vi "EngineeringTool.vi"() -> ()   [LabVIEW 2014]
uses:
  EngineeringGlobals.vi
panel:
  out "Connected":bool
  in  "Close":bool
  in  "Tab Control":enum32{"General", "ARC", "Headers", "Misc"}(tab)
  in  "DSP Code":bool
  in  "Detector":bool
  in  "Temperatures":bool
  in  "Test Shutter":bool
  in  "Manual Commands":bool
  in  "Clear Detector":bool
  in  "Reset Command":bool
  in  "Test Fibers":bool
  in  "Read/Write DSP Memory":bool
  in  "Start Idle Clocks":bool
  in  "Stop Idle Clocks":bool
  in  "Digital I/O":bool
  in  "GetControllerHeader":bool
  in  "GetInstrumentHeader":bool
  in  "GetTelescopeHeader":bool
  out "Server":string
  out "Port":i32
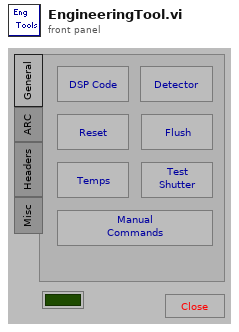
[diagram p1: front panel]
types:
  T1 = typedef "LVRectTypeDef.ctl" = cluster{"Left":i16, "Top":i16, "Right":i16, "Bottom":i16}
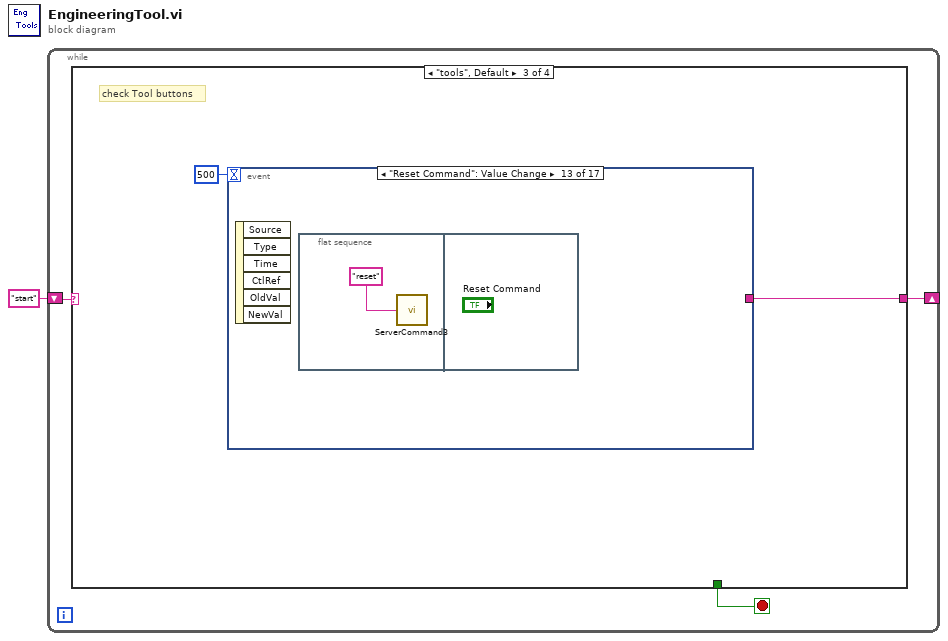
[diagram p0: block diagram]
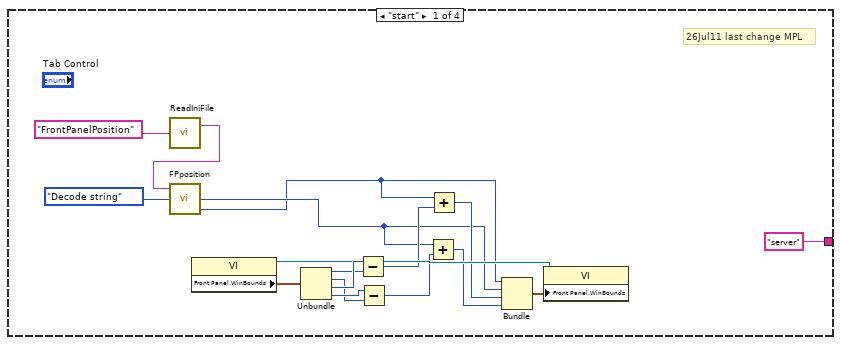
[diagram p2: hidden frame]
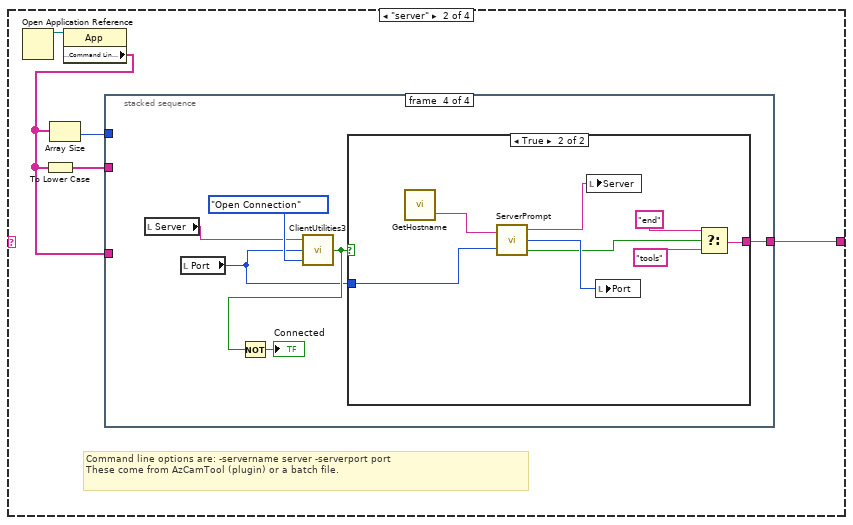
[diagram p3: hidden frame]
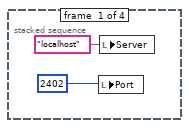
[diagram p4: hidden frame]
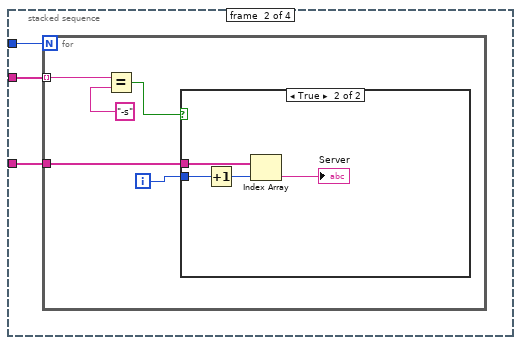
[diagram p5: hidden frame]
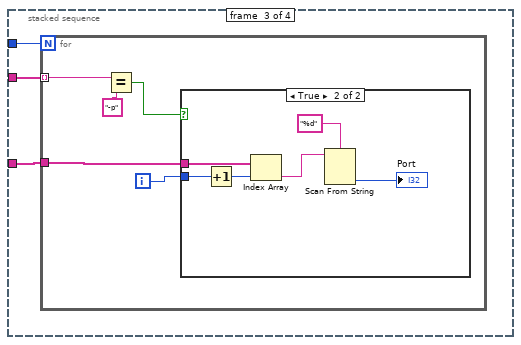
[diagram p7: hidden frame]
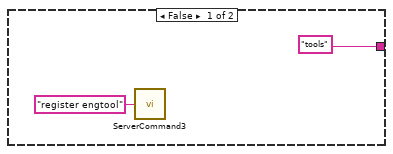
[diagram p9: hidden frame]
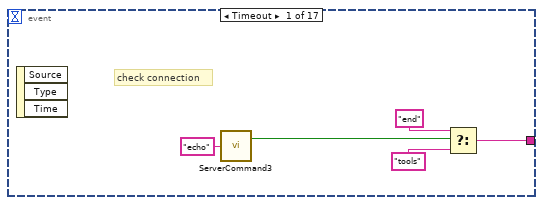
[diagram p10: hidden frame]
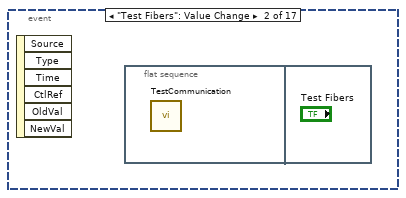
[diagram p11: hidden frame]
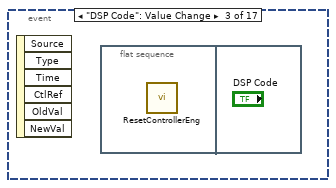
[diagram p12: hidden frame]
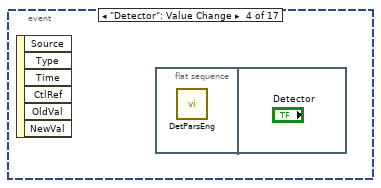
[diagram p13: hidden frame]
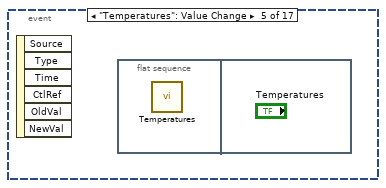
[diagram p14: hidden frame]
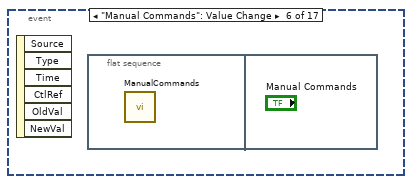
[diagram p15: hidden frame]
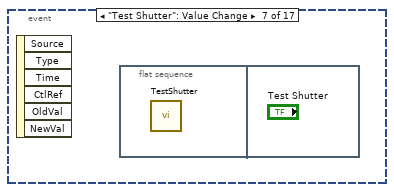
[diagram p16: hidden frame]
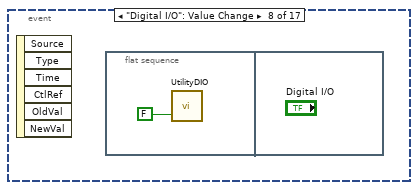
[diagram p17: hidden frame]
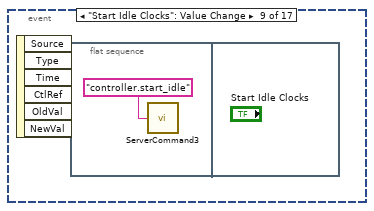
[diagram p18: hidden frame]
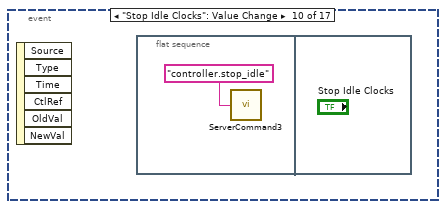
[diagram p19: hidden frame]
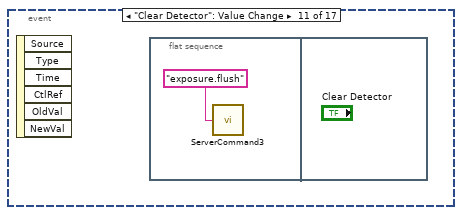
[diagram p20: hidden frame]
diagram:
  n1 = while {
    shift-right: [w3] -> _
    shift-left: "start" -> [w4]
    stop <- w2 stop-if-true
    n2 = case shown="\"tools\", Default" w4 {
      tunnel: ["server" w22 w72 _] -> w3
      tunnel: [_ _ _ TRUE] -> w2
      frame "start" {
        # "26Jul11 last change MPL"
        n3 = call "ReadIniFile.vi"("key"="FrontPanelPosition") -> ("value"=w5:string)  [unwired: 1 out]
        n4 = call "FPposition.vi"("Action"=enum16{"Make string", "Decode string"}."Decode string", "String In"=w5) -> ("left"=w7:i32, "top"=w8:i32)  [unwired: 1 in, 1 out]
        n5 = property class="VI"() -> (reference out=w15:refnum<vi>, "Front Panel.WinBounds"=w20:T1)  [unwired: 2 in, 1 out]
        n6 = Unbundle(w20) -> ("Left"=w18:i16, "Top"=w16:i16, "Right"=w19:i16, "Bottom"=w17:i16)
        n7 = Subtract(x=w19, y=w18) -> (x-y=w11:i16)
        n8 = Subtract(x=w17, y=w16) -> (x-y=w10:i16)
        n9 = Add(x=w8, y=w10) -> (x+y=w12:i32)
        n10 = Add(x=w7, y=w11) -> (x+y=w13:i32)
        n11 = Bundle("left"=w7, "top"=w8, w13, w12) -> (w14:cluster{"left":i32, "top":i32, i32, i32})  [unwired: 1 in]
        n12 = property class="VI"(reference=w15, "Front Panel.WinBounds"=w14) -> ()  [unwired: 1 in, 2 out]
      }
      frame "server" {
        # "Command line options are: -servername server -serverport port\nThese come from AzCamTool (plugin) or a batch file."
        n13 = Open Application Reference() -> (3:w26:refnum<vi>)  [unwired: 4 in, 1 out]
        n14 = property class="App"(reference=w26) -> ("Application:Command Line Arguments"=w24:string[])  [unwired: 1 in, 2 out]
        n15 = To Lower Case(string=w24) -> (all lower case string=w25:string[])
        n16 = Array Size(array=w24) -> (size(s)=w23:i32)
        n17 = stacked-sequence {
          tunnel: w24 -> [_ w30 w42 _]
          tunnel: w25 -> [_ w31 w43 _]
          tunnel: w23 -> [_ w29 w41 _]
          tunnel: [_ _ _ w58] -> w22
          frame #0 {
            n18 = local write "Port"(u16 2402 ("AzCamServer Port")) -> ()
            n19 = local write "Server"("localhost" ("Server")) -> ()
          }
          frame #1 {
            n20 = for {
              N: w29 -> [_]
              tunnel: w31 -> [w34] mode=indexing
              tunnel: w30 -> [w33]
              i -> [w32]
              n21 = Equal?(x=w34, y="-s" ("x")) -> (x = y?=w35:bool)
              n22 = case shown="True" w35 {
                tunnel: w33 -> [_ w39]
                tunnel: w32 -> [_ w38]
                frame False {
                }
                frame True {
                  n23 = Increment(x=w38) -> (x+1=w40:i32)
                  n24 = Index Array(array=w39, index=w40) -> (element=→"Server":string)
                }
              }
            }
          }
          frame #2 {
            n25 = for {
              N: w41 -> [_]
              tunnel: w43 -> [w46] mode=indexing
              tunnel: w42 -> [w45]
              i -> [w44]
              n26 = Equal?(x=w46, y="-p" ("x")) -> (x = y?=w47:bool)
              n27 = case shown="True" w47 {
                tunnel: w45 -> [_ w53]
                tunnel: w44 -> [_ w52]
                frame False {
                }
                frame True {
                  n28 = Increment(x=w52) -> (x+1=w54:i32)
                  n29 = Index Array(array=w53, index=w54) -> (element=w51:string)
                  n30 = Scan From String(format string="%d", input string=w51) -> (output 1=→"Port":i32)  [unwired: 3 in, 3 out]
                }
              }
            }
          }
          frame #3 {
            n31 = local read "Server"() -> (w59:string)
            n32 = local read "Port"() -> (w55:i32)
            n33 = call "ClientUtilities3.vi"("Action"=enum16{"Open Connection"}."Open Connection", "ServerPort"=w55, "ServerName"=w59) -> ("Error"=w57:bool)
            n34 = Not(x=w57) -> (.not. x?=→"Connected":bool)
            n35 = case shown="True" w57 {
              tunnel: ["tools" w65] -> w58
              tunnel: w55 -> [_ w63]
              frame False {
                n36 = call "ServerCommand3.vi"("Command"="register engtool") -> ()  [unwired: 2 out]
              }
              frame True {
                n37 = call "GetHostname.vi"() -> ("Name"=w68:string)  [unwired: 1 in, 1 out]
                n38 = call "ServerPrompt.vi"("AzCam Hostname"=w68, "Port"=w63) -> ("ServerOut"=w70:string, "Port Out"=w69:u16, "Error"=w64:bool)
                n39 = local write "Server"(w70) -> ()
                n40 = local write "Port"(w69) -> ()
                n41 = Select(t="end", s=w64, f="tools") -> (s? t:f=w65:string)
              }
            }
          }
        }
      }
      frame "tools", Default {
        # "check Tool buttons"
        n42 = event shown="[12] \"Reset Command\": Value Change" {
          selector: _ -> [_ _ _ _ _ _ _ _ _ _ _ _ _ _ _ _ _]
          dyn-events: _ -> [_ _ _ _ _ _ _ _ _ _ _ _ _ _ _ _ _]
          timeout: 500 -> [_ _ _ _ _ _ _ _ _ _ _ _ _ _ _ _ _]
          tunnel: [w77 _ _ _ _ _ _ _ _ _ _ _ _ _ _ _ "end"] -> w72
          event Timeout {
            # "check connection"
            n43 = event-data() -> ()  [unwired: 1 in, 3 out]
            n44 = call "ServerCommand3.vi"("Command"="echo") -> ("Error"=w73:bool)  [unwired: 1 out]
            n45 = Select(t="end", s=w73, f="tools") -> (s? t:f=w77:string)
          }
          event "Test Fibers": Value Change {
            n46 = event-data() -> ()  [unwired: 1 in, 6 out]
            n47 = flat-sequence {
              frame #0 {
                n48 = call "TestCommunication.vi"() -> ()  [unwired: 1 in]
              }
              frame #1 {
              }
            }
          }
          event "DSP Code": Value Change {
            n49 = event-data() -> ()  [unwired: 1 in, 6 out]
            n50 = flat-sequence {
              frame #0 {
                n51 = call "ResetControllerEng.vi"() -> ()  [unwired: 1 in, 1 out]
              }
              frame #1 {
              }
            }
          }
          event "Detector": Value Change {
            n52 = event-data() -> ()  [unwired: 1 in, 6 out]
            n53 = flat-sequence {
              frame #0 {
                n54 = call "DetParsEng.vi"() -> ()  [unwired: 2 in]
              }
              frame #1 {
              }
            }
          }
          event "Temperatures": Value Change {
            n55 = event-data() -> ()  [unwired: 1 in, 6 out]
            n56 = flat-sequence {
              frame #0 {
                n57 = call "Temperatures.vi"() -> ()  [unwired: 2 in, 1 out]
              }
              frame #1 {
              }
            }
          }
          event "Manual Commands": Value Change {
            n58 = event-data() -> ()  [unwired: 1 in, 6 out]
            n59 = flat-sequence {
              frame #0 {
                n60 = call "ManualCommands.vi"() -> ()  [unwired: 1 in, 1 out]
              }
              frame #1 {
              }
            }
          }
          event "Test Shutter": Value Change {
            n61 = event-data() -> ()  [unwired: 1 in, 6 out]
            n62 = flat-sequence {
              frame #0 {
                n63 = call "TestShutter.vi"() -> ()  [unwired: 1 in]
              }
              frame #1 {
              }
            }
          }
          event "Digital I/O": Value Change {
            n64 = event-data() -> ()  [unwired: 1 in, 6 out]
            n65 = flat-sequence {
              frame #0 {
                n66 = call "UtilityDIO.vi"("Immediate"=FALSE) -> ()  [unwired: 1 in, 1 out]
              }
              frame #1 {
              }
            }
          }
          event "Start Idle Clocks": Value Change {
            n67 = event-data() -> ()  [unwired: 1 in, 6 out]
            n68 = flat-sequence {
              frame #0 {
                n69 = call "ServerCommand3.vi"("Command"="controller.start_idle") -> ()  [unwired: 2 out]
              }
              frame #1 {
              }
            }
          }
          event "Stop Idle Clocks": Value Change {
            n70 = event-data() -> ()  [unwired: 1 in, 6 out]
            n71 = flat-sequence {
              frame #0 {
                n72 = call "ServerCommand3.vi"("Command"="controller.stop_idle") -> ()  [unwired: 2 out]
              }
              frame #1 {
              }
            }
          }
          event "Clear Detector": Value Change {
            n73 = event-data() -> ()  [unwired: 1 in, 6 out]
            n74 = flat-sequence {
              frame #0 {
                n75 = call "ServerCommand3.vi"("Command"="exposure.flush") -> ()  [unwired: 2 out]
              }
              frame #1 {
              }
            }
          }
          event "Read/Write DSP Memory": Value Change {
            n76 = event-data() -> ()  [unwired: 1 in, 6 out]
            n77 = flat-sequence {
              frame #0 {
                n78 = call "DSPMemory.vi"() -> ()  [unwired: 1 in]
              }
              frame #1 {
              }
            }
          }
          event "Reset Command": Value Change {
            n79 = event-data() -> ()  [unwired: 1 in, 6 out]
            n80 = flat-sequence {
              frame #0 {
                n81 = call "ServerCommand3.vi"("Command"="reset") -> ()  [unwired: 2 out]
              }
              frame #1 {
              }
            }
          }
          event "GetTelescopeHeader": Value Change {
            n82 = event-data() -> ()  [unwired: 1 in, 6 out]
            n83 = flat-sequence {
              frame #0 {
                n84 = call "TelescopeHeader.vi"() -> ()  [unwired: 1 in]
              }
              frame #1 {
              }
            }
          }
          event "GetInstrumentHeader": Value Change {
            n85 = event-data() -> ()  [unwired: 1 in, 6 out]
            n86 = flat-sequence {
              frame #0 {
                n87 = call "InstrumentHeader.vi"() -> ()  [unwired: 1 in]
              }
              frame #1 {
              }
            }
          }
          event "GetControllerHeader": Value Change {
            n88 = event-data() -> ()  [unwired: 1 in, 6 out]
            n89 = flat-sequence {
              frame #0 {
                n90 = call "ControllerHeader.vi"() -> ()  [unwired: 1 in]
              }
              frame #1 {
              }
            }
          }
          event "Close": Value Change {
            n91 = event-data() -> ()  [unwired: 1 in, 6 out]
          }
        }
      }
      frame "end" {
        n92 = stacked-sequence {
          frame #0 {
            n93 = case shown="True" TRUE {
              frame False {
              }
              frame True {
                n94 = call "ServerCommand3.vi"("Command"="CloseConnection()") -> ()  [unwired: 2 out]
              }
            }
          }
          frame #1 {
            n95 = global read "EngineeringGlobals.vi" "ConnectionID 3"() -> (w87:refnum<k5>)
            n96 = TCP Close Connection(connection ID=w87) -> ()  [unwired: 2 in, 2 out]
          }
          frame #2 {
            n97 = property class="VI" props=["Name"]() -> (reference out=w88:refnum<vi>)  [unwired: 2 in, 2 out]
            n98 = call "FPposition.vi"("VI Ref"=w88, "Action"=enum16{"Make string", "Decode string"}."Make string") -> ("String Out"=w89:string)  [unwired: 1 in, 2 out]
            n99 = call "WriteIniFile.vi"("value"=w89, "key"="FrontPanelPosition") -> ()  [unwired: 1 in]
          }
          frame #3 {
            n100 = case shown="True" TRUE {
              frame False {
              }
              frame True {
                n101 = invoke class="VI" method="FP.Close"() -> (reference out=w94:refnum<vi>, error out=w93:errorcluster)  [unwired: 3 in, 1 out]
                n102 = invoke class="VI" method="Abort VI"(reference=w94, error in=w93) -> ()  [unwired: 1 in, 3 out]
              }
            }
          }
        }
      }
    }
  }
